vi "close.vi"(8 "error in":errorcluster, 11 "OPC UA runtime in":refnum<class "OPC UA runtime.lvclass">) -> (0 "error out":errorcluster)   [LabVIEW 2013, in "OPC UA runtime.lvclass"]
doc: "Provides an interface for terminating a module instance. While this interface performs no operations, a child should close and deallocate any open references or memory."
uses:
  OPC UA runtime.lvclass
  OPC UA runtime.lvclass/OPC UA runtime.ctl
  <vilib>/opcua/NI OPC UA Client.lvlib
  <vilib>/opcua/NI OPC UA Server.lvlib
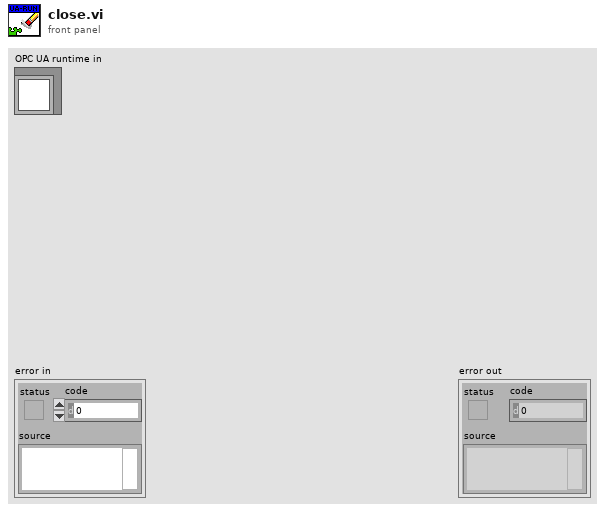
[diagram p1: front panel]
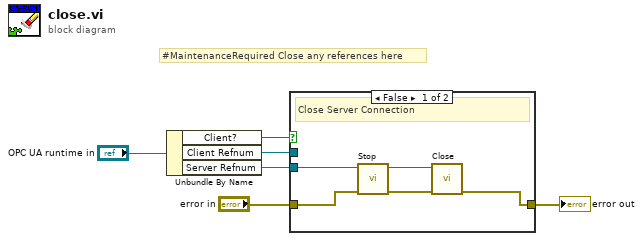
[diagram p0: block diagram]
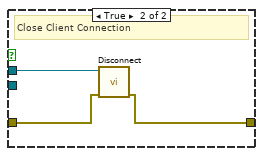
[diagram p2: hidden frame]
diagram:
  # "#MaintenanceRequired Close any references here"
  n1 = Unbundle By Name("OPC UA runtime in") -> ("Client?"=w5:bool, "Client Refnum"=w4:refnum<k21>, "Server Refnum"=w3:refnum<k21>)
  n2 = case shown="False" w5 {
    tunnel: w4 -> [_ w14]
    tunnel: w3 -> [w10 _]
    tunnel: "error in" -> [w8 w13]
    tunnel: [w11 w12] -> w1
    frame False {
      # "Close Server Connection"
      n3 = call <vilib>:"Stop.vi"("error in (no error)"=w8, "OPC UA server refnum in"=w10) -> ("error out"=w7:errorcluster, "OPC UA server refnum out"=w9:refnum<k21>)  [unwired: 8 in]
      n4 = call <vilib>:"Close.vi"("error in (no error)"=w7, "OPC UA server refnum in"=w9) -> ("error out"=w11:errorcluster)  [unwired: 9 in]
    }
    frame True {
      # "Close Client Connection"
      n5 = call <vilib>:"Disconnect.vi"("error in (no error)"=w13, "OPC UA client refnum in"=w14) -> ("error out"=w12:errorcluster)  [unwired: 9 in]
    }
  }
  "error out" <- w1
